vi "Generate mechine code.vi"(0 "DAC default volts 3":dbl[](array[numeric]), 1 "Modules 1":T1(array[cluster]), 2 "Modules 2":T1(array[cluster]), 3 "Modules 3":T1(array[cluster]), 4 "Modules 4":T1(array[cluster]), 5 "Modules 5":T1(array[cluster]), 6 "Modules 6":T1(array[cluster]), 8 "DAC default volts 2":dbl[](array[numeric]), 9 "Section enables":bool[](array[boolean]), 10 "DAC default volts 1":dbl[](array[numeric]), 11 "Durations":string[](array[string])) -> (15 "AO1 times":dbl[](array[numeric]), 16 "Timing data":u64[](array[numeric]), 17 "AO2 times":dbl[](array[numeric]), 18 "Outputs of port A and B":u64[](array[numeric]), 19 "AO3 times":dbl[](array[numeric]), 20 "Outputs of port C and D":u64[](array[numeric]), 21 "max module time":dbl, 22 "AO3":dbl[][](array[numeric]), 23 "AO2":dbl[][](array[numeric]), 24 "AO1":dbl[][](array[numeric]), 25 "Before evap time":dbl, 26 "GPIB output":T2(array[cluster]))   [LabVIEW 2017]
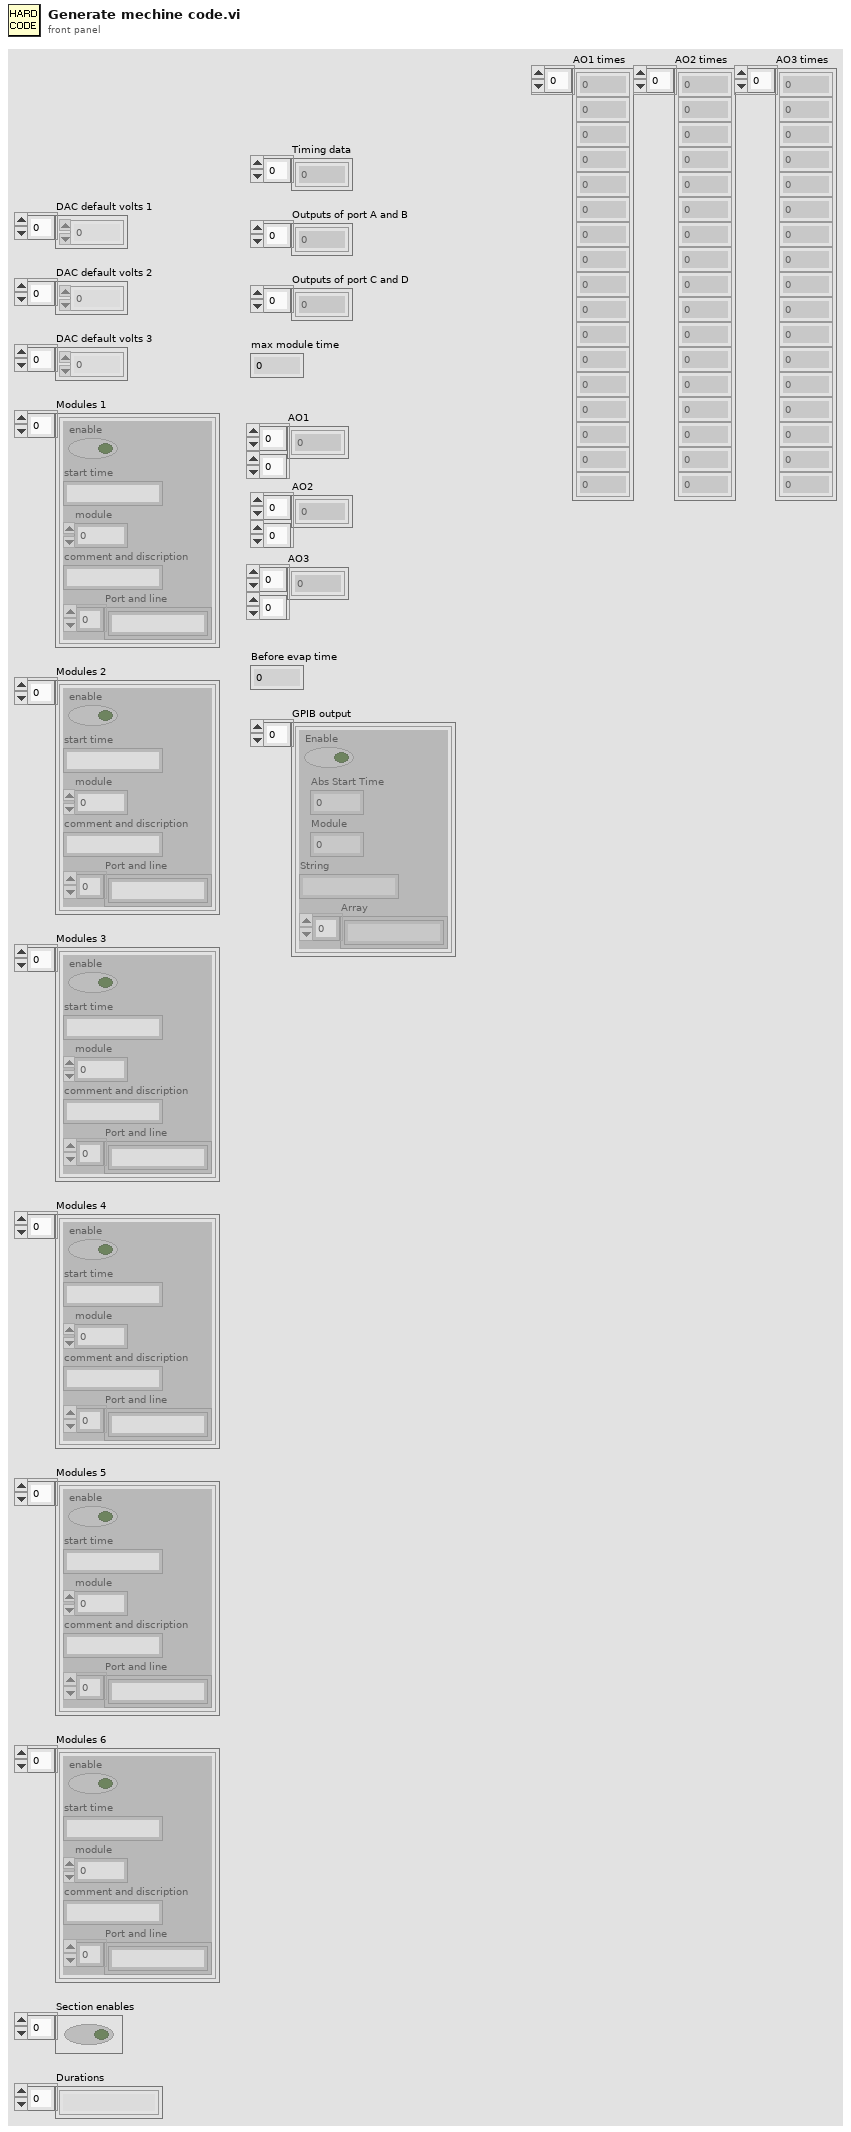
[diagram p1: front panel]
types:
  T1 = cluster{"enable":bool, "start time":string, "module":u16, "comment and discription":string, "Port and line":string[]}[]
  T2 = cluster{"Enable":bool, "Abs Start Time":dbl, "Module":u16, "String":string, "Array":string[]}[]
  T3 = cluster{"Times":dbl[], "Voltages":dbl[], "Enable Ch":bool, "Hinge Points":u8}[]
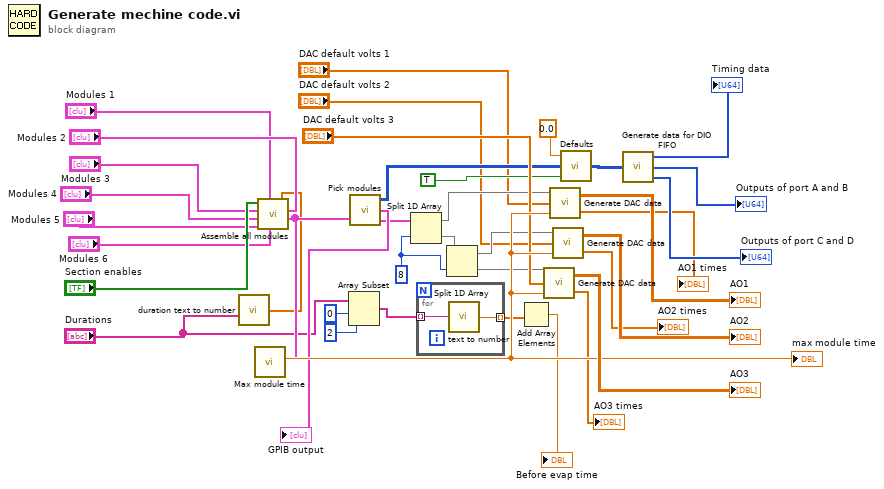
[diagram p0: block diagram]
diagram:
  w34 = 8 ("index")
  n1 = call "duration text to number.vi"("durations (ms)"="Durations") -> ("durations2 (ms)"=w5:dbl[])
  n2 = call "Assemble all modules.vi"("Module List 2"="Modules 2", "durations"=w5, "Module List 6"="Modules 6", "Module List 1"="Modules 1", "Module List 5"="Modules 5", "Module List 4"="Modules 4", "Module List 3"="Modules 3", "Module Enabled Array"="Section enables") -> ("Module Array"=w17:T2)  [unwired: 1 out]
  n3 = call "Max module time.vi"("Module Array"=w17) -> ("max value"=w38:dbl)  [unwired: 10 in]
  "max module time" <- w38
  n4 = Array Subset(array="Durations", index=0, length=2) -> (w19:string[])
  n5 = call "Pick modules.vi"("Module List"=w17) -> ("Output Data"=w27:i64[][], "GPIB output"=→"GPIB output":T2, "Static output"=w6:T3)  [unwired: 1 in]
  n6 = Split 1D Array(array=w6, index=w34) -> (first subarray=w26:T3, second subarray=w33:T3)
  n7 = for {
    tunnel: w19 -> [w41] mode=indexing
    tunnel: [w40] -> w18 mode=indexing
    n8 = call "text to number.vi"("text"=w41) -> ("number"=w40:dbl)
  }
  n9 = Split 1D Array(array=w33, index=w34) -> (first subarray=w35:T3, second subarray=w36:T3)
  n10 = Add Array Elements(numeric array=w18) -> (sum=→"Before evap time":dbl)
  n11 = call "Generate DAC data.vi"("End time"=w38, "Default voltages"="DAC default volts 3", "Input Array"=w36) -> ("times"=→"AO3 times":dbl[], "Output"=→"AO3":dbl[][])
  n12 = call "Generate DAC data.vi"("End time"=w38, "Default voltages"="DAC default volts 1", "Input Array"=w26) -> ("times"=→"AO1 times":dbl[], "Output"=→"AO1":dbl[][])
  n13 = call "Generate DAC data.vi"("End time"=w38, "Default voltages"="DAC default volts 2", "Input Array"=w35) -> ("times"=→"AO2 times":dbl[], "Output"=→"AO2":dbl[][])
  n14 = call "Defaults.vi"("Do this?"=TRUE, "Input"=w27, "Absolute start time (ms)"=0.0) -> ("Output"=w23:i64[][])
  n15 = call "Generate data for DIO FIFO.vi"("Times, Ports, Lines, Values"=w23) -> ("Outputs of port C and D"=→"Outputs of port C and D":u64[], "Outputs of port A and B"=→"Outputs of port A and B":u64[], "Timing data"=→"Timing data":u64[])  [unwired: 2 in]
